vi "s-lab第6章 数据类型转换1-11.vi"() -> ()   [LabVIEW 2013]
panel:
  out "数值 3":dbl
  in  "布尔 4":bool
  out "数组 6":bool[](array[boolean])
  in  "数值 2":dbl
  in  "布尔 3":bool
  out "数字":u32
  in  "布尔 2":bool
  in  "布尔":bool
  out "数组 5":dbl[](array[numeric])
  in  "簇 2":cluster{"旋钮":dbl, "数值":dbl} {"旋钮" scale=0.0..10.0}
  out "簇":T1
  in  "数组 4":dbl[](array[knob]) scale=0.0..10.0
  out "数组 3":u32[](array[numeric]) format="%x"
  in  "十六进制字符串":string
  out "字符串 2":string
  in  "数组 2":dbl[](array[numeric])
  out "数组":i32[](array[numeric]) format="%x"
  out "字符串":string
  out "十六进制字符串转为十进制数值":dbl
  out "十进制数值":dbl
  in  "十六进制字符串":string
  in  "十进制字符串":string
  in  "小数点后位数":dbl
  out "数值":dbl
  in  "旋钮":dbl(knob) scale=0.0..10.0
  out "格式字符串":string
  out "十六进制字符串":string
  out "十进制字符串":string
  in  "十进制数值2":dbl
  in  "十进制数值1":dbl
  out "路径字符串":string
  in  "路径输入":path
  out "路径":path
  in  "输入路径字符串":string
  # "例 1"
  # "例 2"
  # "注意：路径选择时必须指定路径下的一个文件，但转换后的字符串中不包含该文件名。\n         可以手动输入路径，手动输入时最后一个“\\”符号被自动删除。"
  # "例 3"
  # "注意：小数点位数后的数据显示为4舍5入。当小数点后均为0时就不受位数限制了，\n         能显示6位，如：10.000000"
  # "例 4"
  # "注意：字符串显示控件必须选择“十六进制”显示，否则显示汉字或乱码。\n         \n         数组显示控件不能选择“十六进制”显示，所以只能显示十进制数。\n         将数值显示控件的显示类型由“DBL”改为整形，然后“十六进制”            \n         显示即可选择。\n\n         转换后的字符串显示为两个一组，中间有空格，实际上中间没有空\n         格字符。"
  # "例 5"
  # "例 6"
  # "注意：字符串显示控件必须选择“十六进制”显示，否则显示ascII码。"
  # "例 7"
  # "注意：簇必须由“数组至簇转换”控件创建，否则出错。自动创建的簇里\n         面有8个数值显示控件，删掉任何一个都会出错，原因不明。\n原因：因为放置的是“旋钮”控件，数组 4中最多包含8个给类型元素，\n         在创建该数组时将余下的全部创建出来了。"
  # "例 8"
  # "例 9"
  # "例 10"
  # "例 11"
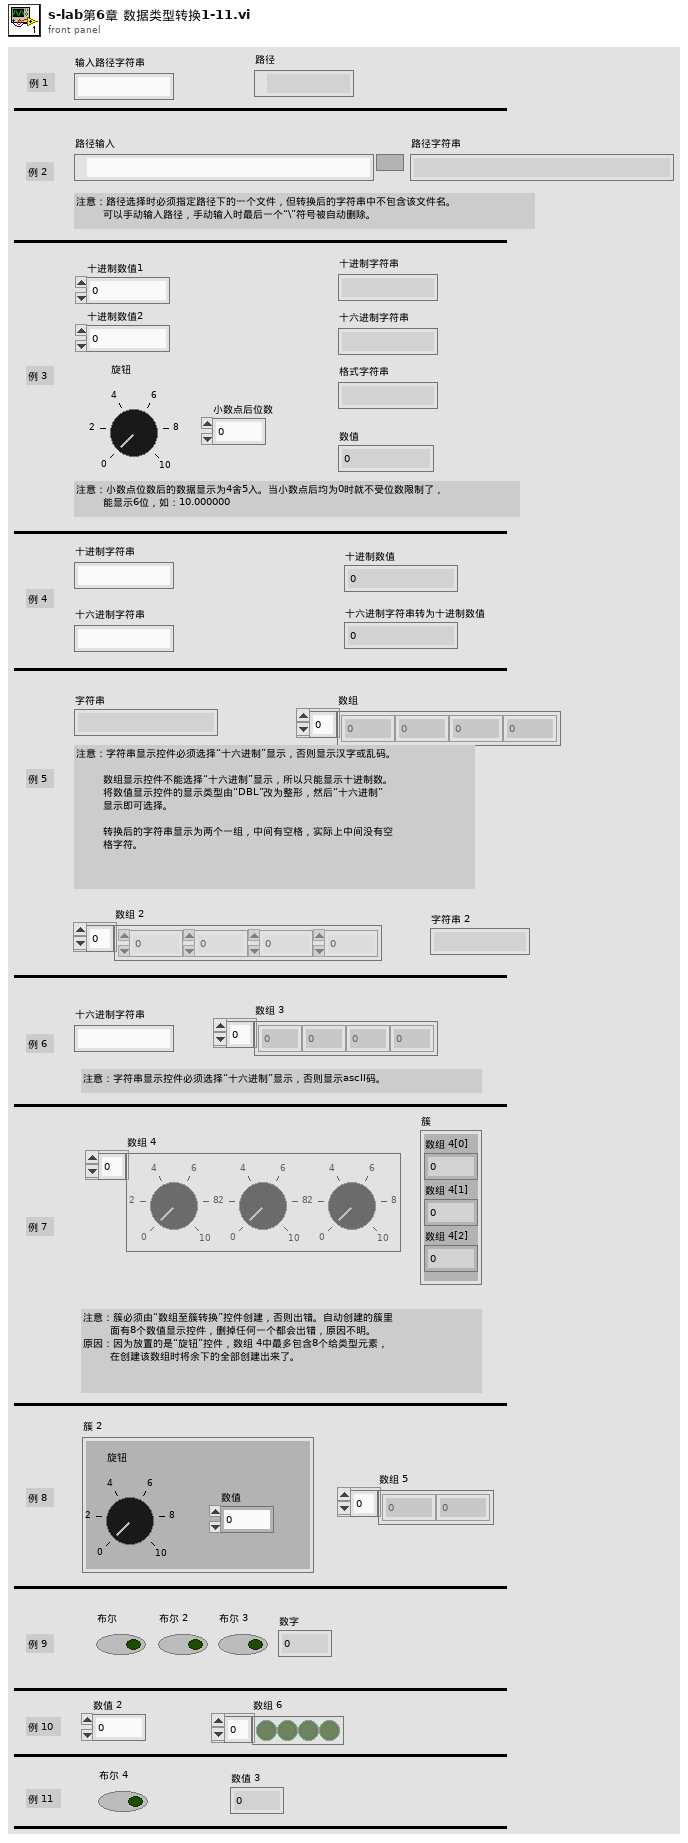
[diagram p1: front panel]
types:
  T1 = cluster{"数组 4[0]":dbl, "数组 4[1]":dbl, "数组 4[2]":dbl, "数组 4[3]":dbl, "数组 4[4]":dbl, "数组 4[5]":dbl, "数组 4[6]":dbl, "数组 4[7]":dbl, "数组 4[8]":dbl}
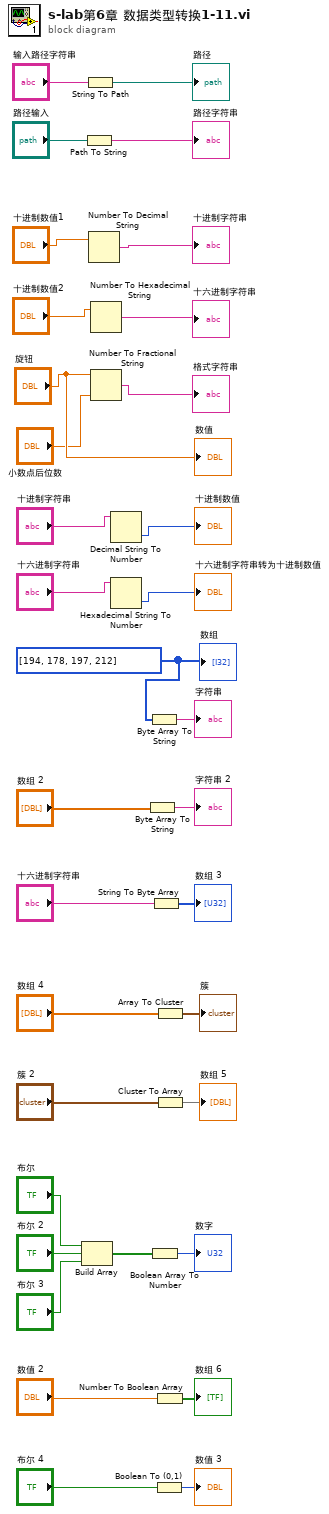
[diagram p0: block diagram]
diagram:
  w18 = i32[] [194, 178, 197, 212]
  n1 = Build Array("布尔", "布尔 2", "布尔 3") -> (w7:bool[])
  n2 = Path To String(path="路径输入") -> (string=→"路径字符串":string)
  n3 = String To Path(string="输入路径字符串") -> (path=→"路径":path)
  n4 = Number To Decimal String(number="十进制数值1") -> (decimal integer string=→"十进制字符串":string)  [unwired: 1 in]
  n5 = Number To Hexadecimal String(2:"十进制数值2") -> (0:→"十六进制字符串":string)  [unwired: 1 in]
  n6 = Number To Fractional String(number="旋钮", precision (6)="小数点后位数") -> (F-format string=→"格式字符串":string)  [unwired: 2 in]
  n7 = Decimal String To Number(string="十进制字符串") -> (number=→"十进制数值":i32)  [unwired: 2 in, 1 out]
  n8 = Hexadecimal String To Number(string="十六进制字符串") -> (number=→"十六进制字符串转为十进制数值":u32)  [unwired: 2 in, 1 out]
  n9 = Byte Array To String(unsigned byte array="数组 2") -> (string=→"字符串 2":string)
  n10 = Byte Array To String(unsigned byte array=w18) -> (string=→"字符串":string)
  n11 = Boolean Array To Number(Boolean array=w7) -> (number=→"数字":u32)
  n12 = String To Byte Array(string="十六进制字符串") -> (unsigned byte array=→"数组 3":u8[])
  n13 = Boolean To (0,1)(Boolean="布尔 4") -> (0, 1=→"数值 3":i16)
  n14 = Array To Cluster(array="数组 4") -> (cluster=→"簇":T1)
  n15 = Cluster To Array(cluster="簇 2") -> (array=→"数组 5":dbl[])
  n16 = Number To Boolean Array(number="数值 2") -> (Boolean array=→"数组 6":bool[])
  "数值" <- "旋钮"
  "数组" <- w18
